vi "读取数值.vi"(8 "error in (no error)":errorcluster, 10 "Slave ID":u8=1, 11 "MB session in":refnum<class "MB_Master.lvclass">) -> (0 "error out":errorcluster, 2 "读取值":T1, 3 "MB session out":refnum<class "MB_Master.lvclass">)   [LabVIEW 2016, in "流量计集成.lvlib" / "LSS-10Q博亿达流量计.lvlib"]
uses:
  <vilib>/Plasmionique/MB Master/MB_Master/MB_Master.lvclass
  <vilib>/Plasmionique/MB Master/MB Master.lvlib
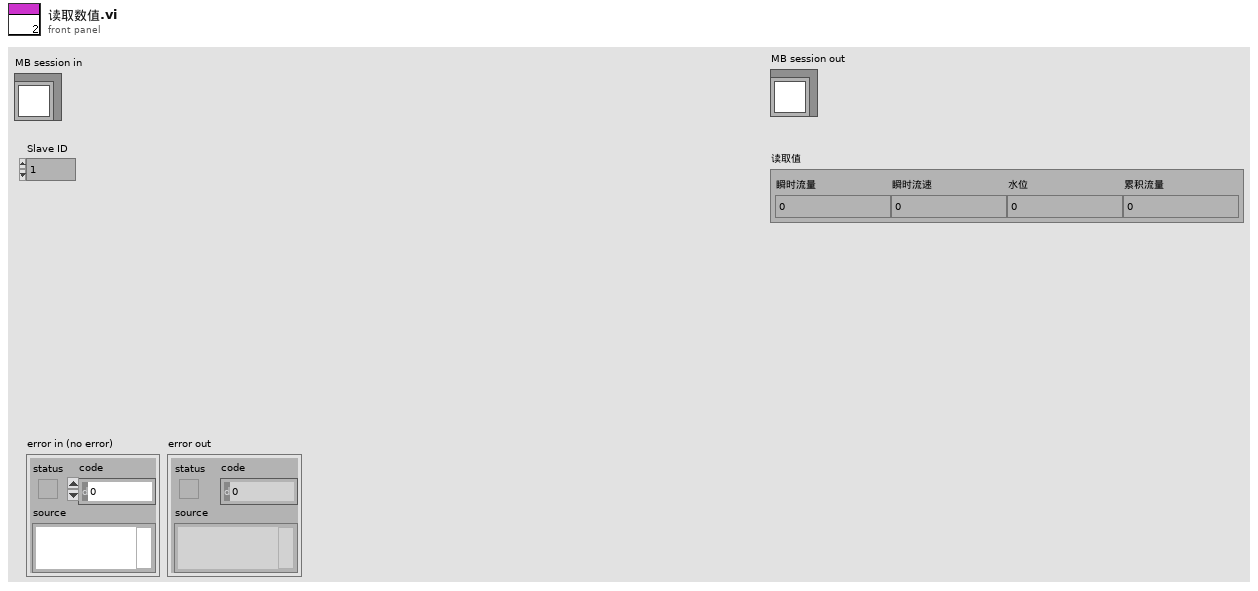
[diagram p1: front panel]
types:
  T1 = typedef "流量计集成.lvlib/博意达流量计.lvlib/读取值.ctl" = cluster{"瞬时流量":sgl, "瞬时流速":sgl, "水位":sgl, "累积流量":sgl}
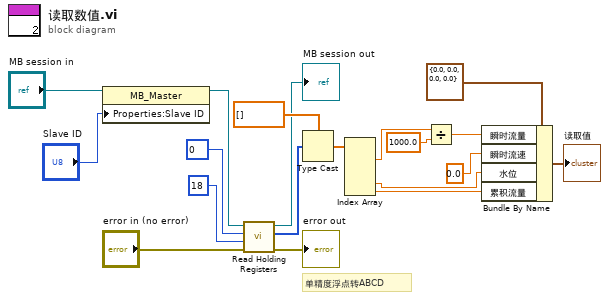
[diagram p0: block diagram]
diagram:
  # "单精度浮点转ABCD"
  n1 = property class="MB_Master"(reference="MB session in", "Properties:Slave ID"="Slave ID") -> (reference out=w17:refnum<class "MB_Master.lvclass">)  [unwired: 1 in, 1 out]
  n2 = call <vilib>:"Read Holding Registers.vi"("error in (no error)"="error in (no error)", "quantity"=u16 18, "starting address"=u16 0, "MB session in"=w17) -> ("error out"=→"error out":errorcluster, "Registers"=w18:u16[], "MB session out"=→"MB session out":refnum<class "MB_Master.lvclass">)  [unwired: 5 in]
  n3 = Type Cast(type=sgl[] [], x=w18) -> (*(type *) &x=w9:sgl[])
  n4 = Index Array(array=w9) -> (element #1=w7:sgl, element #4=w4:sgl, element #5=w3:sgl)  [unwired: 5 in, 2 out]
  n5 = Divide(x=w7, y=sgl 1000.0) -> (x/y=w8:sgl)
  n6 = Bundle By Name(cluster=T1 {"瞬时流量"=0.0, "瞬时流速"=0.0, "水位"=0.0, "累积流量"=0.0} ("读取值"), "瞬时流量"=w8, "瞬时流速"=sgl 0.0, "水位"=w4, "累积流量"=w3) -> (→"读取值":T1)
